vi "Create.vi"(9 "Current":string, 10 "Input":string) -> (3 "Proto":refnum<class "Numeric Keypad.lvclass">)   [LabVIEW 2020, in "Numeric Keypad.lvclass"]
uses:
  Numeric Keypad.lvclass
  Numeric Keypad.lvclass/Numeric Keypad.ctl
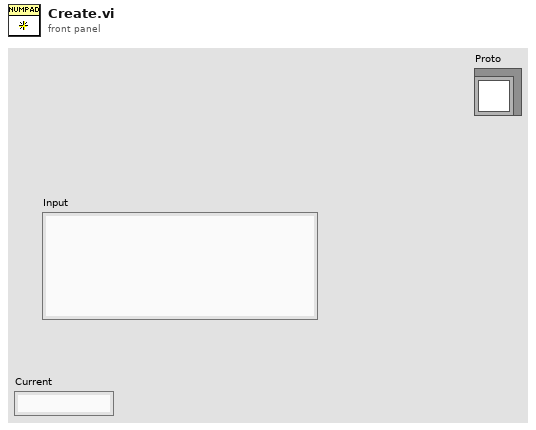
[diagram p1: front panel]
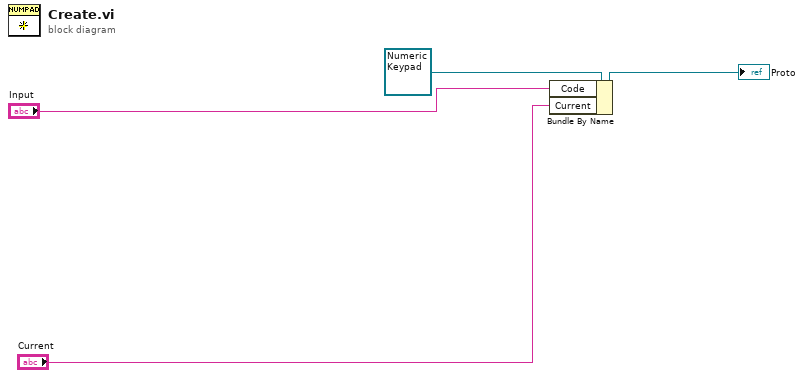
[diagram p0: block diagram]
diagram:
  n1 = Bundle By Name(cluster=refnum<class "Numeric Keypad.lvclass"> refnum ("Proto"), "Code"="Input", "Current"="Current") -> (→"Proto":refnum<class "Numeric Keypad.lvclass">)
